vi "Beam-Breaker-In.vi"() -> (2 "PASSED-IN?":bool, 3 "Counter":dbl)   [LabVIEW 2019]
uses:
  Robot Global Data.vi
  <vilib>/Rock Robotics/SystemInterfaces/DIO/FPGA_DIOChannel.ctl
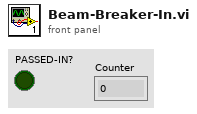
[diagram p1: front panel]
types:
  T1 = typedef "WPI_DigitalOutputDevRef.ctl" = cluster{"DIO Channel":T2, "DevStatus":errorcluster}
  T2 = typedef "FPGA_DIOChannel.ctl" = enum8{"DIO 0", "DIO 1", "DIO 2", "DIO 3", "DIO 4", "DIO 5", "DIO 6", "DIO 7", "DIO 8", "DIO 9", "DIO MXP 0", "DIO MXP 1", "DIO MXP 2", "DIO MXP 3", "DIO MXP 4", "DIO MXP 5", "DIO MXP 6", "DIO MXP 7", "DIO MXP 8", "DIO MXP 9", "DIO MXP 10", "DIO MXP 11", "DIO MXP 12", "DIO MXP 13", "DIO MXP 14", "DIO MXP 15", "SPI Port CS1", "SPI Port CS2", "SPI Port CS3", "SPI Port MISO", "SPI Port MOSI", "Invalid"}
  T3 = typedef "WPI_DigitalInputDevRef.ctl" = cluster{"DevStatus":errorcluster, "DIO Channel":T2}
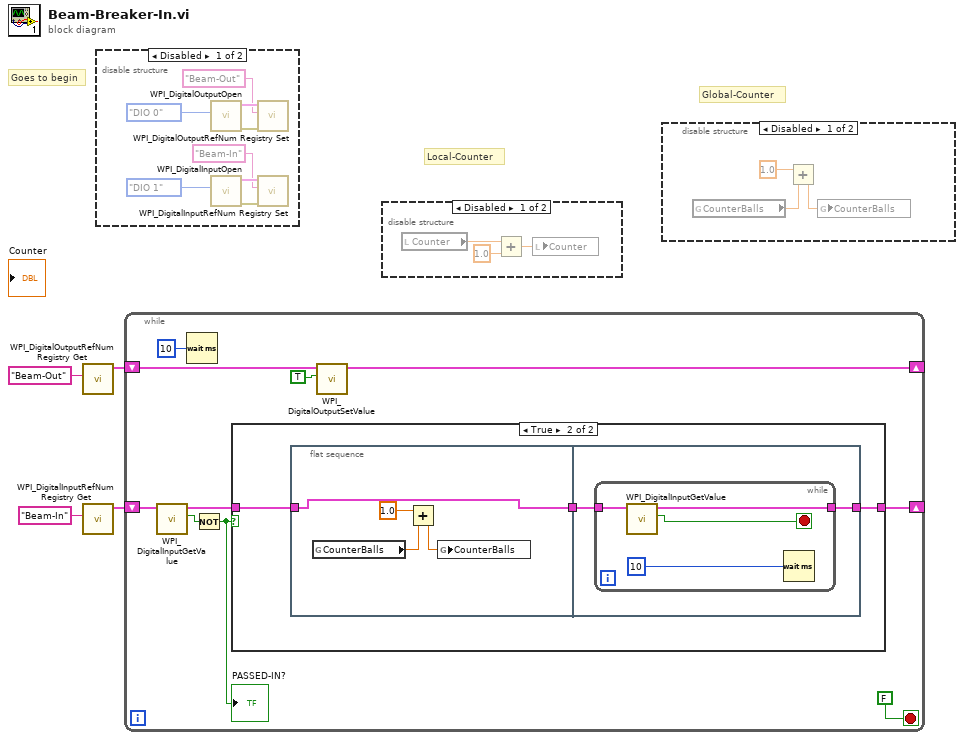
[diagram p0: block diagram]
diagram:
  # "Global-Counter"
  # "Local-Counter"
  # "Goes to begin"
  n1 = call <vilib>:"WPI_DigitalOutputRefNum Registry Get.vi"("refnum name"="Beam-Out") -> ("DigitalOutputDevRef"=w2:T1)  [unwired: 9 in, 1 out]
  n2 = call <vilib>:"WPI_DigitalInputRefNum Registry Get.vi"("refnum name"="Beam-In") -> ("DigitalInputDevRef"=w3:T3)  [unwired: 9 in, 1 out]
  n3 = disable-structure shown="Disabled" {
    frame Disabled {
      n4 = call <vilib>:"WPI_DigitalOutputOpen.vi"("DIO Channel"=FPGA_DIOChannel."DIO 0") -> ("error out"=w5:errorcluster, "DigitalOutputDevRef"=w7:T1)  [unwired: 9 in]
      n5 = call <vilib>:"WPI_DigitalInputOpen.vi"("DIO Channel"=FPGA_DIOChannel."DIO 1") -> ("error out"=w10:errorcluster, "DigitalInputDevRef"=w12:T3)  [unwired: 9 in]
      n6 = call <vilib>:"WPI_DigitalOutputRefNum Registry Set.vi"("error in (no error)"=w5, "refnum name"="Beam-Out", "DigitalOutputDevRef"=w7) -> ()  [unwired: 7 in, 2 out]
      n7 = call <vilib>:"WPI_DigitalInputRefNum Registry Set.vi"("error in (no error)"=w10, "refnum name"="Beam-In", "DigitalInputDevRef"=w12) -> ()  [unwired: 7 in, 2 out]
    }
    frame Enabled {
    }
  }
  n8 = while {
    shift-right: [w19] -> _
    shift-left: w3 -> [w22]
    shift-right: [w17] -> _
    shift-left: w2 -> [w18]
    stop <- FALSE stop-if-true
    n9 = call <vilib>:"WPI_DigitalInputGetValue.vi"("DigitalInputDevRef"=w22) -> ("Value"=w14:bool, "DigitalInputDevRef"=w20:T3)  [unwired: 8 in, 1 out]
    n10 = Wait (ms)(milliseconds to wait=u32 10 ("millisecond timer value")) -> ()  [unwired: 1 out]
    n11 = Not(x=w14) -> (.not. x?=w13:bool)
    "PASSED-IN?" <- w13
    n12 = case shown="True" w13 {
      tunnel: w20 -> [w23 w25]
      tunnel: [w23 w26] -> w19
      frame False {
      }
      frame True {
        n13 = flat-sequence {
          tunnel: w25 -> [w30]
          tunnel: [w30] -> w24
          tunnel: [w32] -> w26
          tunnel: w24 -> [w31]
          frame #0 {
            n14 = global read "Robot Global Data.vi" "CounterBalls"() -> (w27:dbl)
            n15 = Add(x=1.0, y=w27) -> (x+y=w28:dbl)
            n16 = global write "Robot Global Data.vi" "CounterBalls"(w28) -> ()
          }
          frame #1 {
            n17 = while {
              tunnel: w31 -> [w35]
              tunnel: [w34] -> w32
              stop <- w33 stop-if-true
              n18 = call <vilib>:"WPI_DigitalInputGetValue.vi"("DigitalInputDevRef"=w35) -> ("Value"=w33:bool, "DigitalInputDevRef"=w34:T3)  [unwired: 8 in, 1 out]
              n19 = Wait (ms)(milliseconds to wait=u32 10) -> ()  [unwired: 1 out]
            }
          }
        }
      }
    }
    n20 = call <vilib>:"WPI_DigitalOutputSetValue.vi"("Value"=TRUE, "DigitalOutputDevRef"=w18) -> ("DigitalOutputDevRef"=w17:T1)  [unwired: 8 in, 1 out]
  }
  n21 = disable-structure shown="Disabled" {
    frame Disabled {
      n22 = local read "Counter"() -> (w39:dbl)
      n23 = Add(x=w39, y=1.0) -> (x+y=w38:dbl)
      n24 = local write "Counter"(w38) -> ()
    }
    frame Enabled {
    }
  }
  n25 = disable-structure shown="Disabled" {
    frame Disabled {
      n26 = global read "Robot Global Data.vi" "CounterBalls"() -> (w40:dbl)
      n27 = Add(x=1.0, y=w40) -> (x+y=w41:dbl)
      n28 = global write "Robot Global Data.vi" "CounterBalls"(w41) -> ()
    }
    frame Enabled {
    }
  }
